vi "GPS显示界面.vi"() -> ()   [LabVIEW 2016, in "环境动力监测库.lvlib" / "NMEA.lvlib"]
uses:
  NMEA.lvlib
  NMEA_GPVTG-data.ctl
  NMEA_Mode.ctl
  NMEA_GPRMC-data.ctl
  NMEA_LatitudeDirection.ctl
  NMEA_LongitudeDirection.ctl
  NMEA_GPGGA-data.ctl
  NMEA_GPS-Quality.ctl
  <vilib>/Utility/miscctls.llb/LVPointTypeDef.ctl
  <vilib>/Utility/config.llb/NI_LVConfig.lvlib
panel:
  in  "解除告警":bool
  out "x+1":u32
  out "浮标定位点":cluster{"纬度":dbl, "经度":dbl} {"经度" format="%#.6g"; "纬度" format="%#.6g"}
  out "Port":string
  out "IP":string
  in  "手动设置定位":bool caption="定位自动获取OFF/手动设置ON"
  out "波特率":u32
  out "串口":string
  in  "移位报警设定值":dbl=1000.0
  out "GPS-Quality":T1
  out "定位状态":bool=TRUE
  in  "配置":bool
  out "Coordinates":picture
  in  "reset odometer":bool
  out "方位角 (deg)":dbl(knob) scale=0.0..360.0
  out "偏移量/米":dbl format="%#.2f"
  out "水平运动速度 (km/h)":dbl(knob) scale=0.0..180.0
  out "海拔":dbl format="%.2f"
  out "纬度":dbl format="%#.6g"
  out "经度":dbl format="%#.6g"
  out "时间":timestamp format="%<%H:%M:%S>T"
  out "日期":timestamp format="%<%Y/%m/%d>T"
  out "$GPGGA-message_OUT":T2={"TimeStamp"=timestamp(0 s since 1904-01-01), "Latitude"=0.0, "Latitude-Direction"=enum."", "Longitude"=1.0, "Longitude-Direction"=enum."", "GPS-Quality"=enum."GPS fix (SPS)", "Number of Satellites"=0, "Horizontal Dilution of Precision"=0.0, "Altitude above Mean-Sea-Level"=0.0, "Geoidal separation"=0.0, "Time since last DGPS update"=0.0, "DGPS reference station ID"=0} {"Time since last DGPS update" format="%.02f [s]"; "Geoidal separation" format="%.02f [m]"; "Altitude above Mean-Sea-Level" format="%.02f [m]"; "Horizontal Dilution of Precision" format="%.02f [HDOP]"; "Longitude" format="%0.4f [long]"; "Latitude" format="%.04f [lat]"; "TimeStamp" format="%<%.2X>T"}
  out "$GPRMC-message_OUT":T5={"TimeStamp"=timestamp(0 s since 1904-01-01), "Validity"=FALSE, "Latitude"=0.0, "Latitude-Direction"=enum."North", "Longitude"=0.0, "Longitude-Direction"=enum."East", "Speed in knots"=0.0, "True course"=0.0, "Date Stamp"=timestamp(0 s since 1904-01-01), "Magnetic Variation (East/West)"=0.0} {"Magnetic Variation (East/West)" format="%.02f [deg]"; "Date Stamp" format="%<%x>T"; "True course" format="%.02f [deg]"; "Speed in knots" format="%.02f [kts]"; "Longitude" format="%0.4f [long]"; "Latitude" format="%.04f [lat]"; "TimeStamp" format="%<%.2X>T"}
  out "$GPVTG-message_OUT":T6={"True Course over Ground"=0.0, "Magnetic Course over Ground"=0.0, "Speed over Ground in knots"=0.0, "Speed over Ground in km/h"=1.0, "Mode"=""} {"Speed over Ground in km/h" format="%.02f [km/h]"; "Speed over Ground in knots" format="%.02f [kts]"; "Magnetic Course over Ground" format="%.02f [deg]"; "True Course over Ground" format="%.02f [deg]"}
  out "Raw data GPS":string
  # "米"
  # "GPS监测"
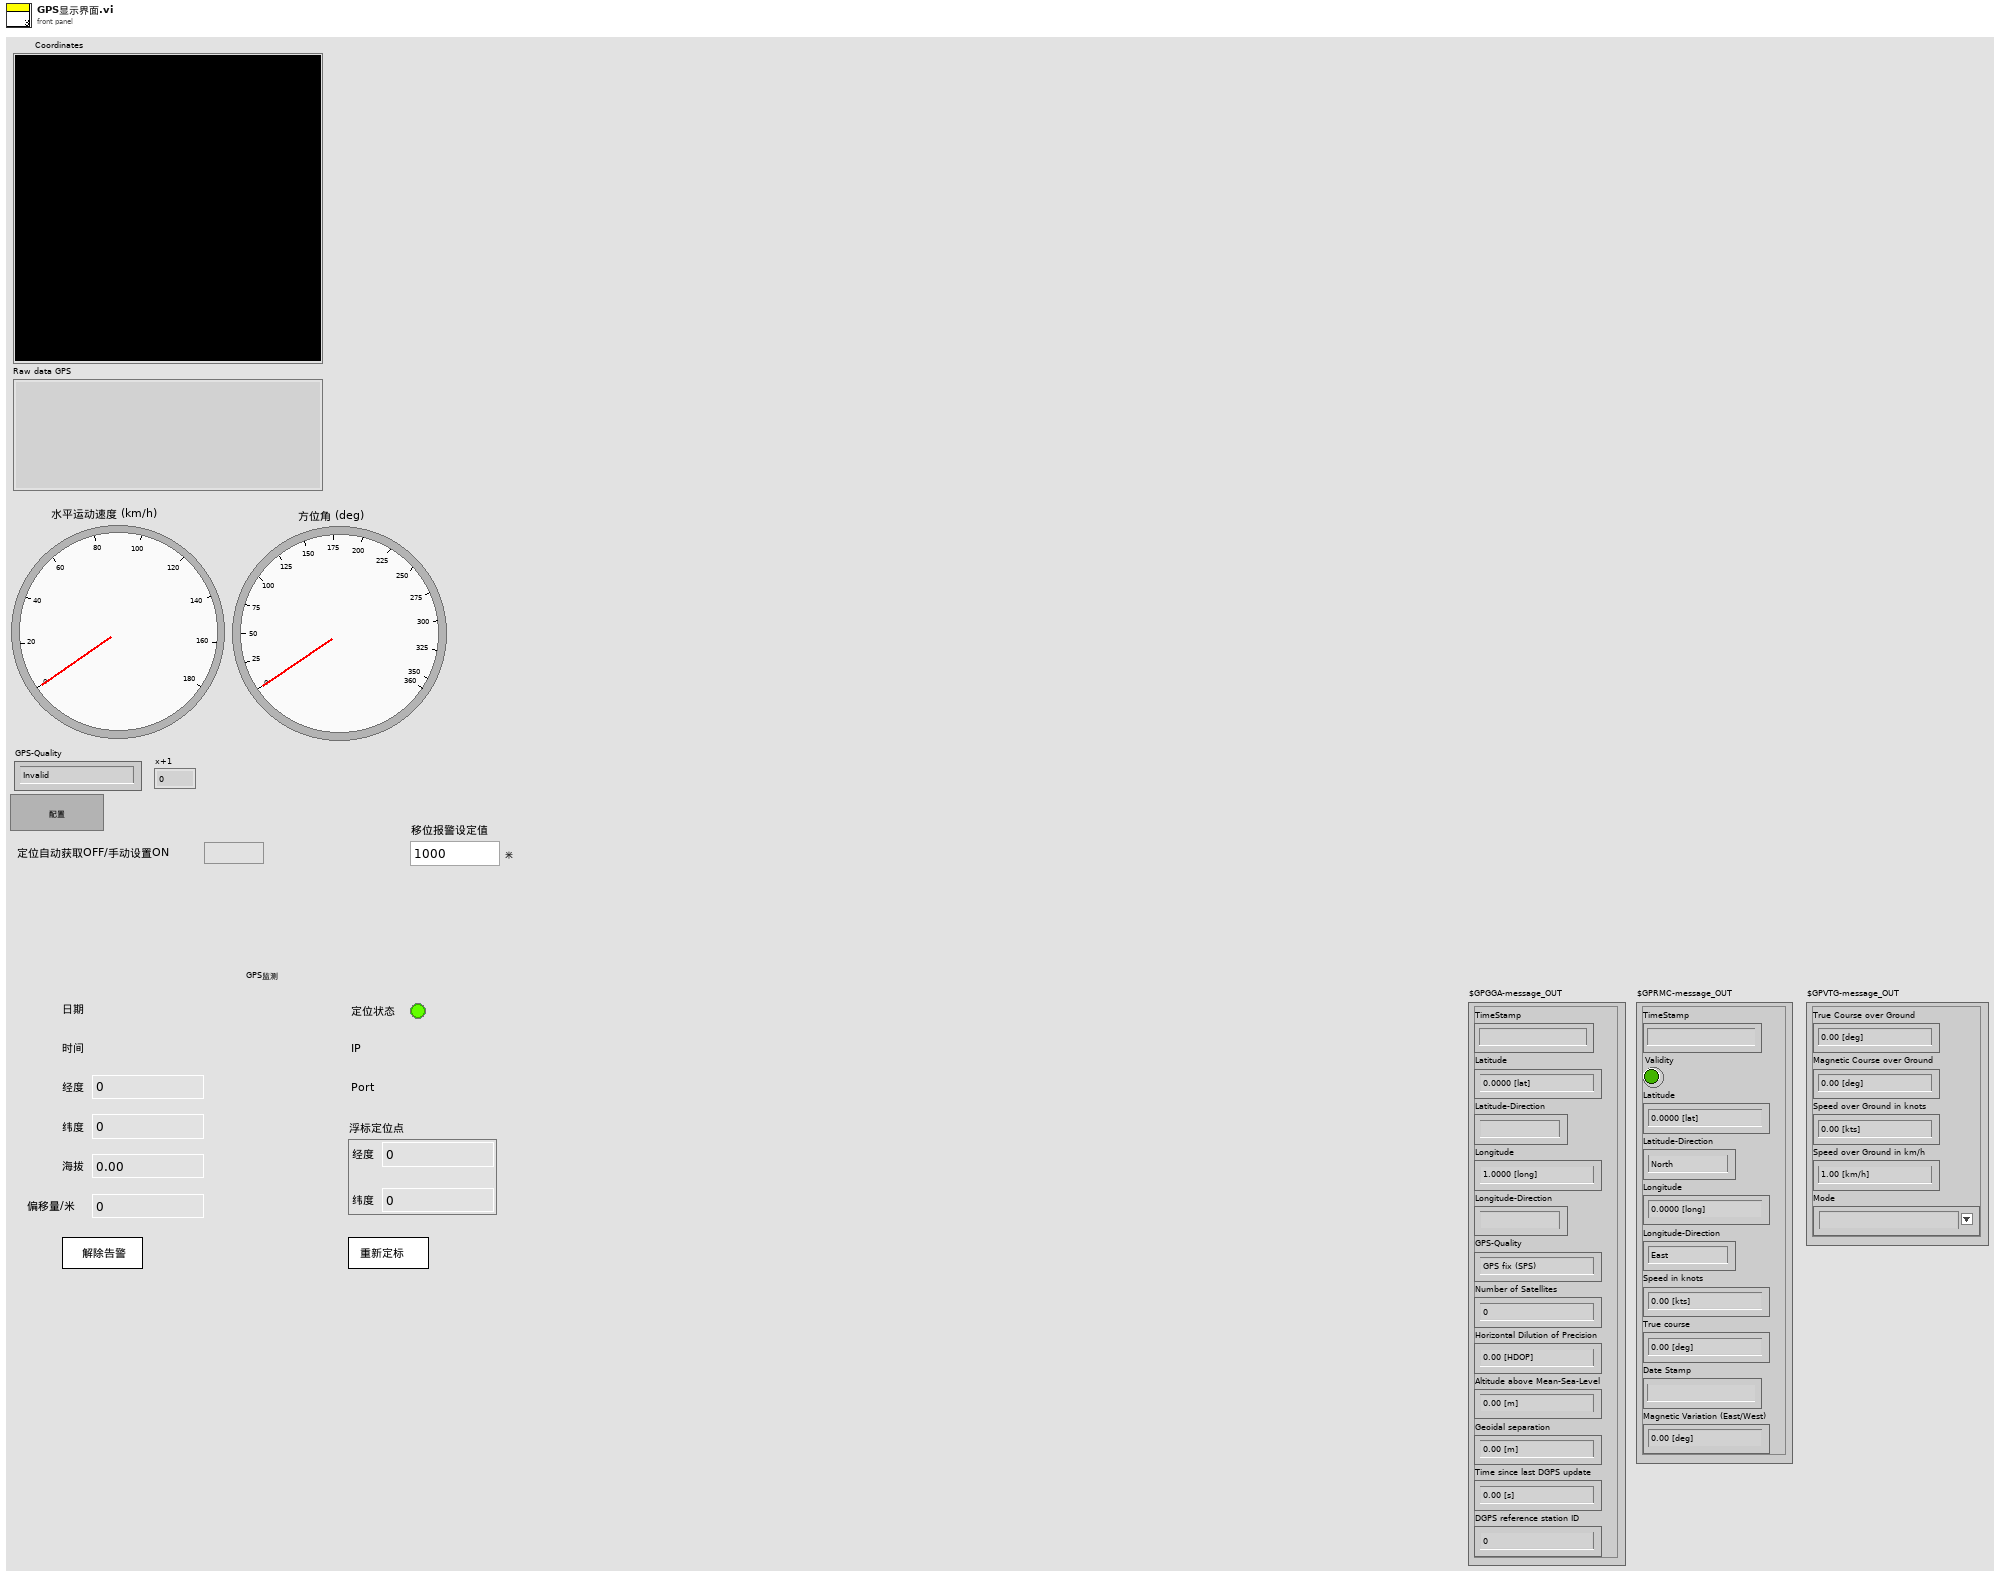
[diagram p1: front panel]
types:
  T1 = typedef "环境动力监测库.lvlib/NMEA.lvlib/NMEA_GPS-Quality.ctl" = enum16{"Invalid", "GPS fix (SPS)", "DGPS fix", "PPS fix", "Real Time Kinematic", "Float RTK", "estimated", "Manual input mode", "Simulation mode"}
  T2 = typedef "环境动力监测库.lvlib/NMEA.lvlib/NMEA_GPGGA-data.ctl" = cluster{"TimeStamp":timestamp, "Latitude":dbl, "Latitude-Direction":T3, "Longitude":dbl, "Longitude-Direction":T4, "GPS-Quality":T1, "Number of Satellites":i32, "Horizontal Dilution of Precision":dbl, "Altitude above Mean-Sea-Level":dbl, "Geoidal separation":dbl, "Time since last DGPS update":dbl, "DGPS reference station ID":i32}
  T3 = typedef "环境动力监测库.lvlib/NMEA.lvlib/NMEA_LatitudeDirection.ctl" = enum16{"", "North", "South"}
  T4 = typedef "环境动力监测库.lvlib/NMEA.lvlib/NMEA_LongitudeDirection.ctl" = enum16{"", "East", "West"}
  T5 = typedef "环境动力监测库.lvlib/NMEA.lvlib/NMEA_GPRMC-data.ctl" = cluster{"TimeStamp":timestamp, "Validity":bool, "Latitude":dbl, "Latitude-Direction":T3, "Longitude":dbl, "Longitude-Direction":T4, "Speed in knots":dbl, "True course":dbl, "Date Stamp":timestamp, "Magnetic Variation (East/West)":dbl}
  T6 = typedef "环境动力监测库.lvlib/NMEA.lvlib/NMEA_GPVTG-data.ctl" = cluster{"True Course over Ground":dbl, "Magnetic Course over Ground":dbl, "Speed over Ground in knots":dbl, "Speed over Ground in km/h":dbl, "Mode":T7}
  T7 = typedef "环境动力监测库.lvlib/NMEA.lvlib/NMEA_Mode.ctl" = string
  T8 = cluster{"监测项描述:输出":string, "连接方式":enum16{"串口", "TCP"}, "端口":string, "IP address:":string, "Port:":string, "站号":u64, "传感器型号":string, "波特率":u64, "data bits":u64, "停止位":u16, "奇偶校验":u16, "声光告警启用":bool}
  T9 = typedef "LVPointTypeDef.ctl" = cluster{"Horizontal":i16, "Vertical":i16}
  T10 = cluster{"定位状态":bool, "卫星数量":u16, "时间标识":timestamp, "纬度":dbl, "南北":string, "经度":dbl, "东西":string}
  T11 = cluster{"网络参数":cluster{"网络状态":bool, "本机IP":string[]}, "电源管理":cluster{"电源管理":bool, "氨氮电源":bool, "总磷电源":bool, "总氮电源":bool, "多参数电源":bool, "CODMn电源":bool, "CODCr电源":bool, "灯带电源":bool, "照明电源":bool}, "北斗-GPS":cluster{"GPS":cluster{"经度:":sgl, "纬度: ":sgl, "GPS监测":bool}, "北斗":cluster{"经度:":sgl, "纬度:":sgl, "北斗监测":bool}}}
  T12 = typedef "NI_LVConfig.lvlib/Config Data RefNum.ctl" = refnum<k1>
  T13 = cluster{"漏水监测输出":cluster{"漏水监测告警":bool, "告警内容":string}, "门禁监测输出":cluster{"门禁监测告警":bool, "告警内容":string}, "门禁监测输出2":cluster{"门禁监测告警":bool, "告警内容":string}, "温湿度监测输出":cluster{"温湿度监测告警":bool, "告警内容":string}, "烟雾监测输出":cluster{"烟雾监测告警":bool, "告警内容":string}, "空调监测输出":cluster{"空调监测告警":bool, "告警内容":string}, "自动重合闸输出":cluster{"自动重合闸告警":bool, "告警内容":string}, "红外入侵输出":cluster{"红外入侵告警":bool, "告警内容":string}, "振动输出":cluster{"振动告警":bool, "告警内容":string}, "UPS输出":cluster{"UPS告警":bool, "告警内容":string}, "蓄电池输出":cluster{"蓄电池告警":bool, "告警内容":string}, "蓄电池输出2":cluster{"蓄电池告警":bool, "告警内容":string}, "GPS输出":cluster{"定位告警":bool, "告警内容":string}, "北斗输出":cluster{"定位告警":bool, "告警内容":string}, "气象输出":cluster{"气象告警":bool, "告警内容":string}}
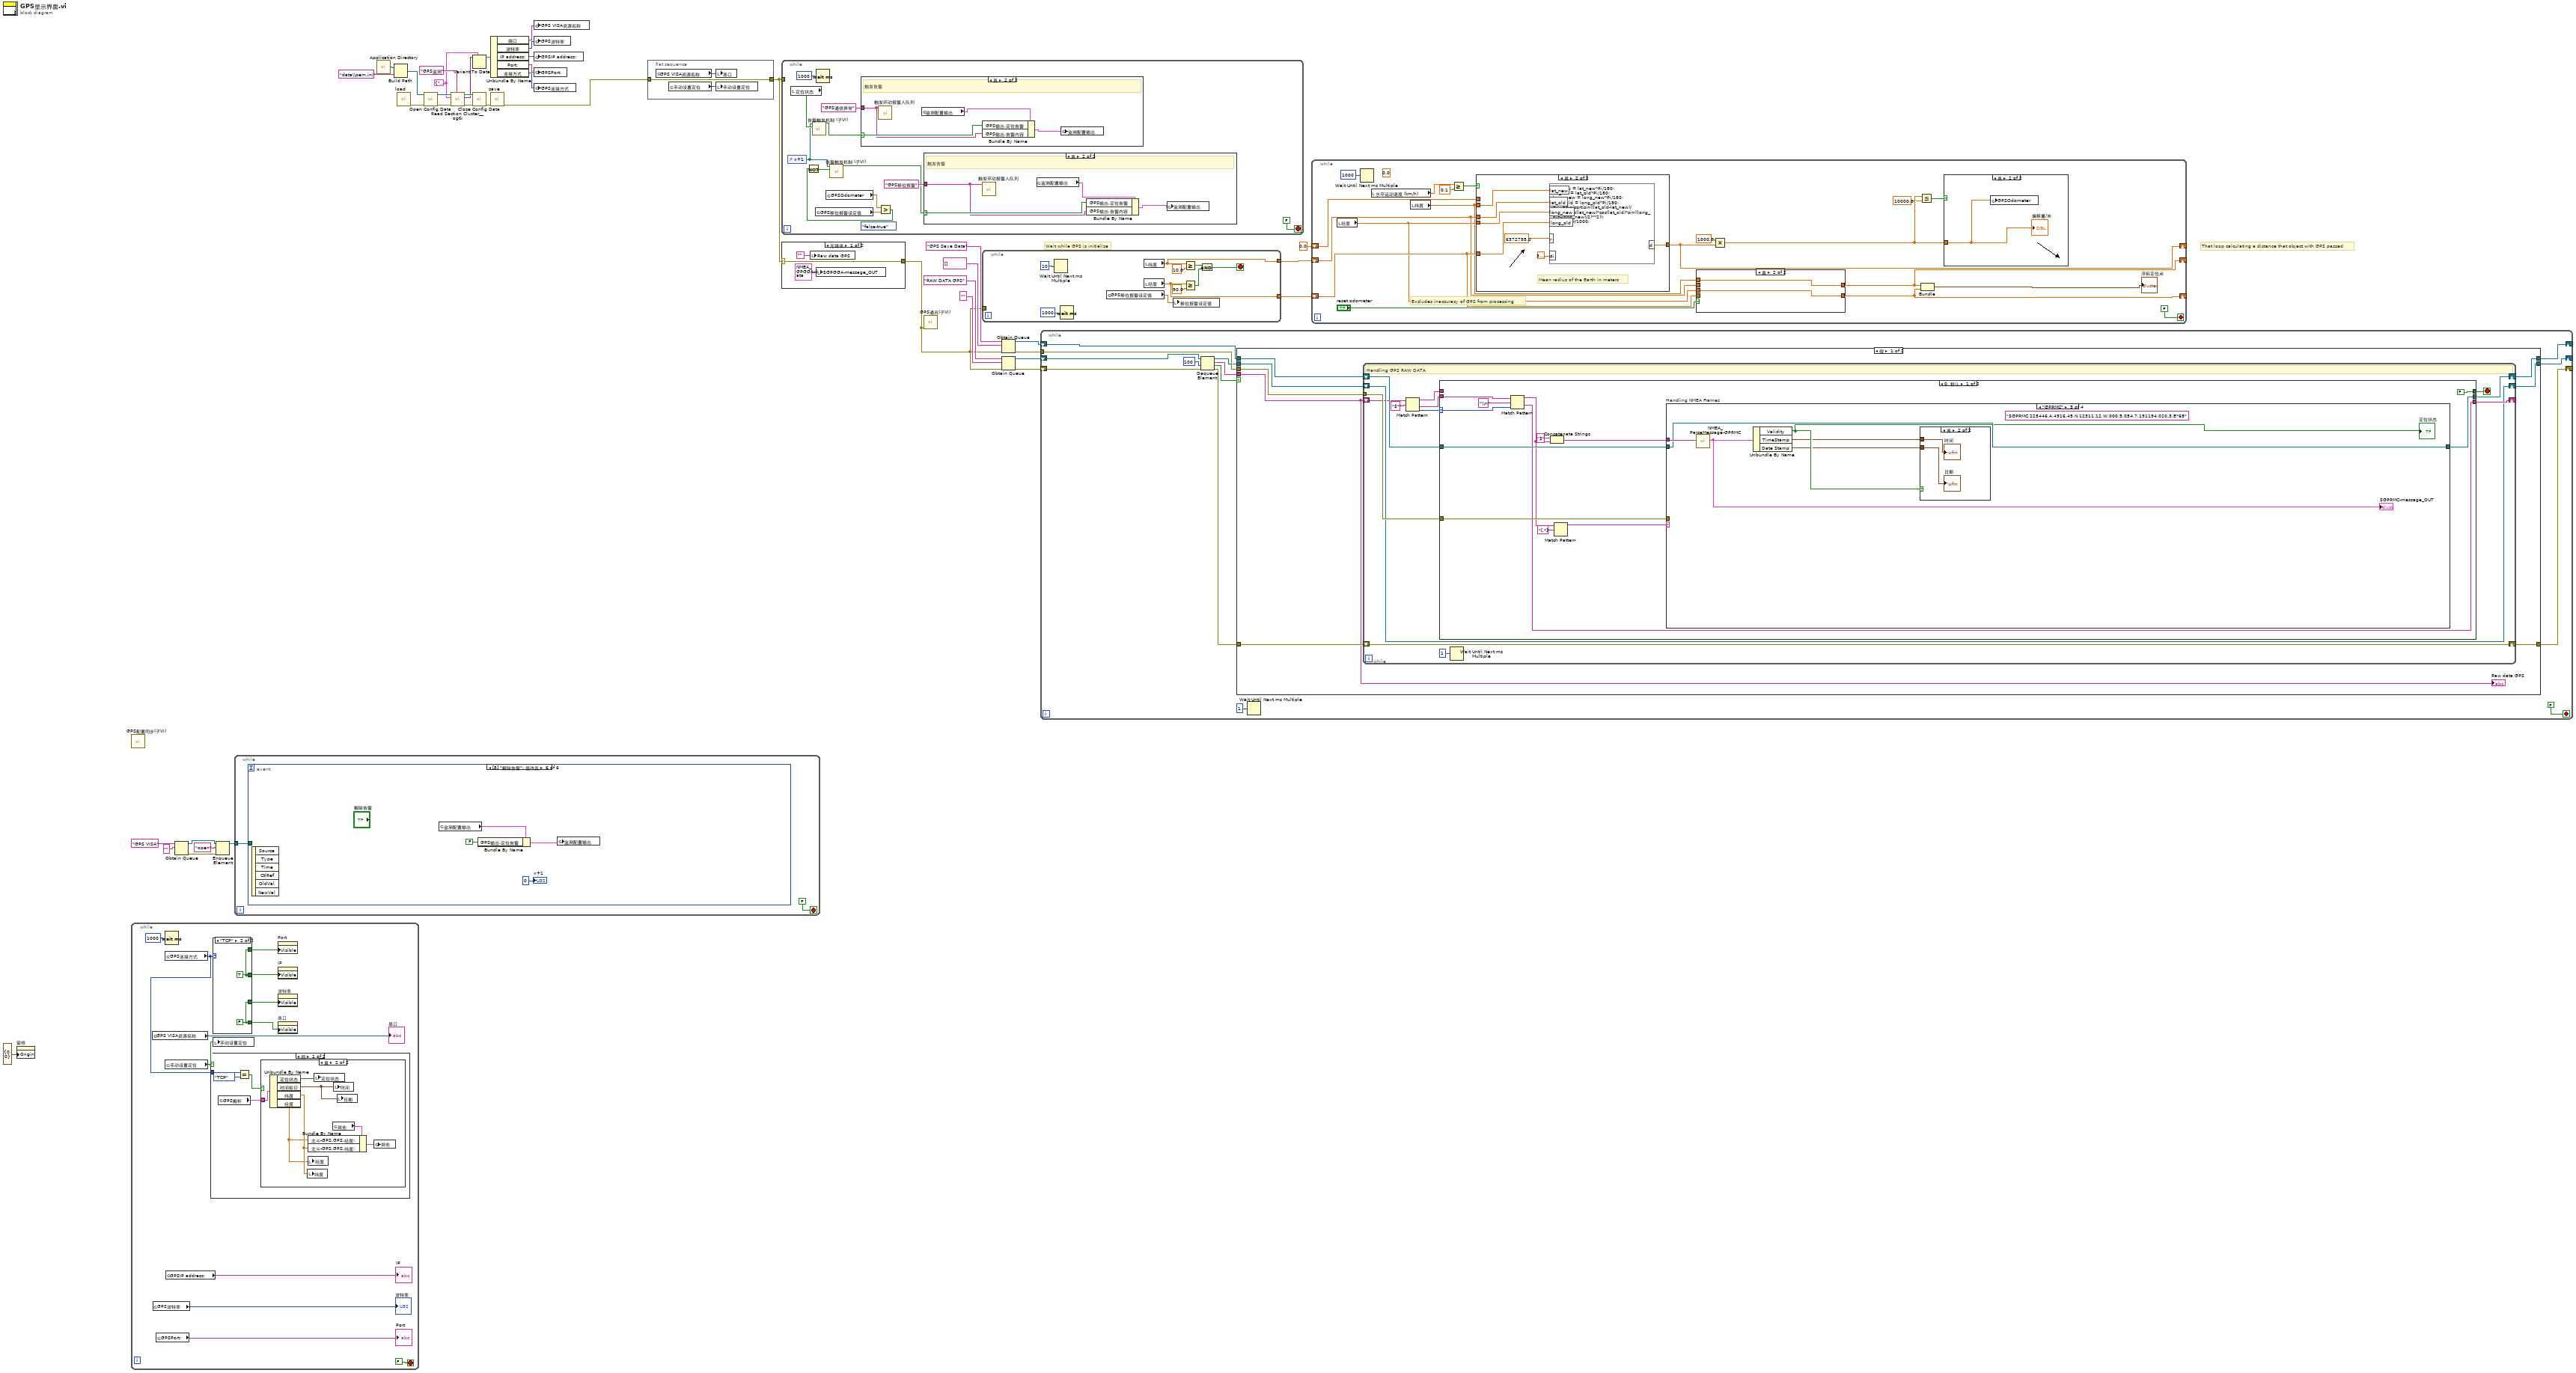
[diagram p0: block diagram]
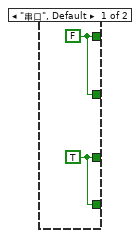
[diagram p4: hidden frame]
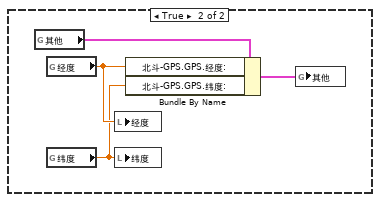
[diagram p6: hidden frame]
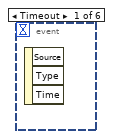
[diagram p7: hidden frame]
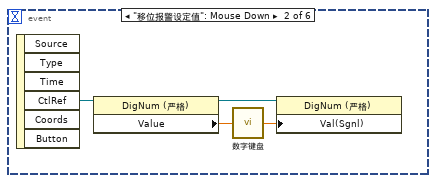
[diagram p8: hidden frame]
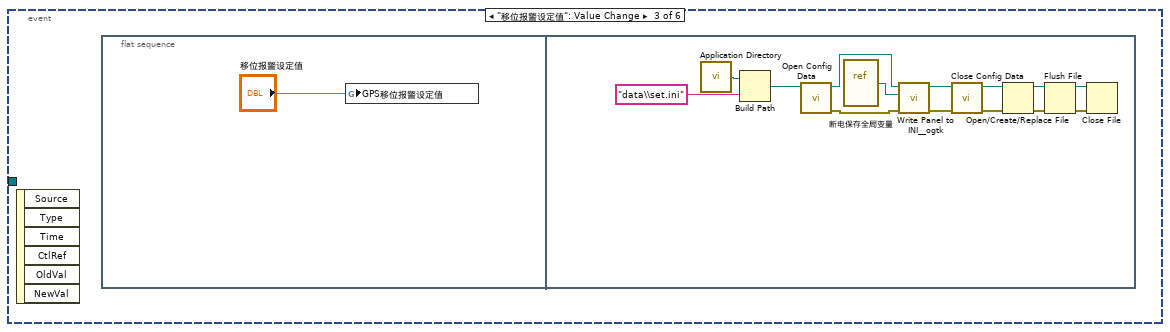
[diagram p9: hidden frame]
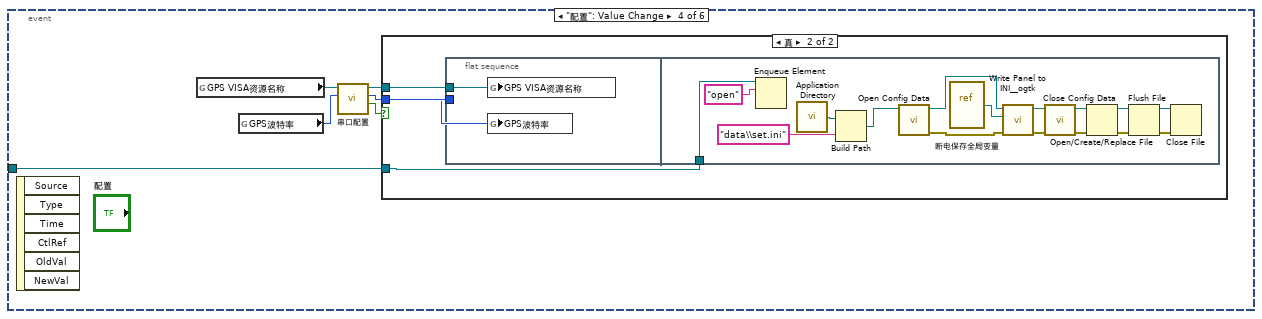
[diagram p10: hidden frame]
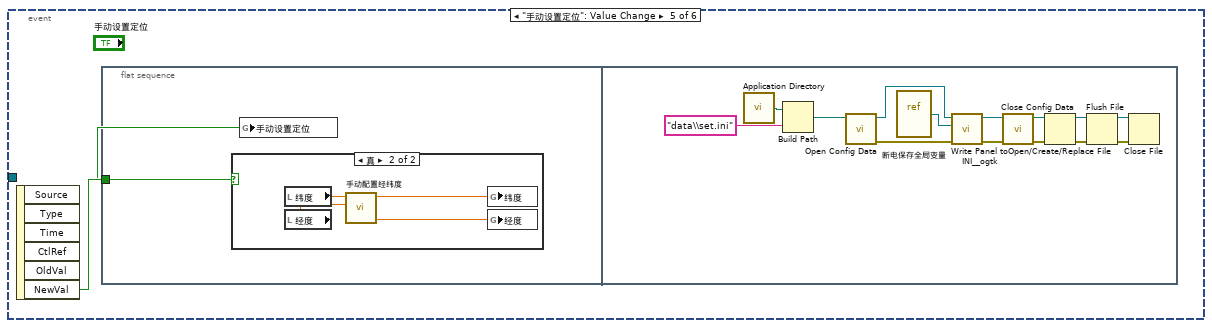
[diagram p12: hidden frame]
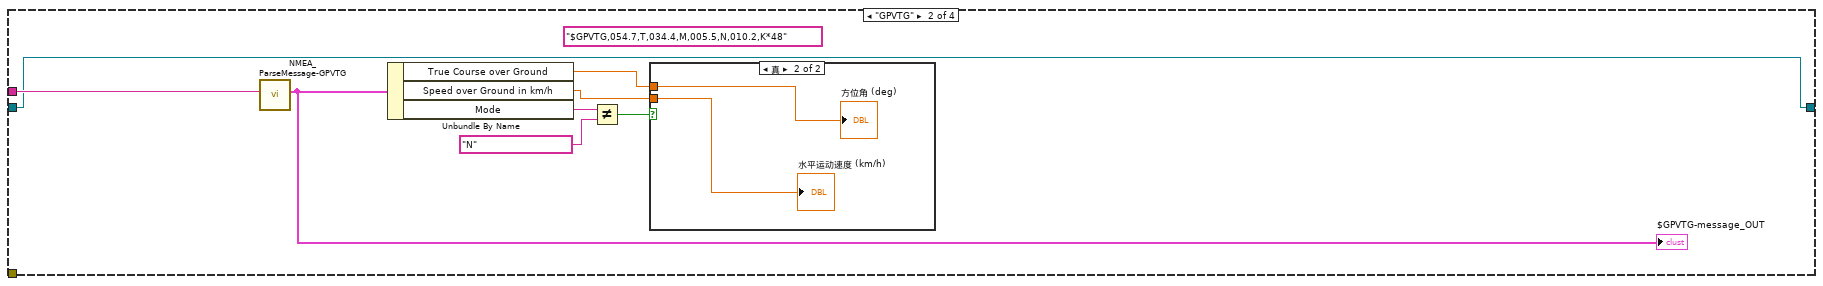
[diagram p19: hidden frame]
diagram:
  w9 = T8 {"监测项描述:输出"="", "连接方式"=enum."串口", "端口"="", "IP address:"="", "Port:"="", "站号"=19200, "传感器型号"="", "波特率"=19200, "data bits"=8, "停止位"=10, "奇偶校验"=0, "声光告警启用"=FALSE} ("输入簇")
  (unwired) 0.0 ("方位角 (deg)")
  # "That loop calculating a distance that object with GPS passed"
  # "Wait while GPS is initialize"
  n1 = property on="窗格" class="Pane"("Origin"=T9 {"Horizontal"=0, "Vertical"=0} ("原点")) -> ()  [unwired: 2 in, 2 out]
  n2 = call "GPS配置同步(子VI).vi"() -> ()  [unwired: 12 in]
  n3 = while {
    stop <- FALSE stop-if-true
    n4 = global read "断电保存全局变量.vi" "GPS VISA资源名称"() -> (→"串口":refnum<visa-resource-name>)
    n5 = global read "断电保存全局变量.vi" "GPS波特率"() -> (→"波特率":u32)
    n6 = global read "断电保存全局变量.vi" "GPSPort:"() -> (→"Port":string)
    n7 = Wait (ms)(milliseconds to wait=u32 1000 ("等待时间（毫秒）")) -> ()  [unwired: 1 out]
    n8 = global read "断电保存全局变量.vi" "GPS连接方式"() -> (w40:enum16{"串口", "TCP"})
    n9 = global read "断电保存全局变量.vi" "手动设置定位"() -> (w47:bool)
    n10 = global read "断电保存全局变量.vi" "GPSIP address:"() -> (→"IP":string)
    n11 = case shown="假" w47 {
      tunnel: w40 -> [w59 _]
      frame False {
        n12 = global read "NMEA过程全局变量.vi" "GPS解析"() -> (w56:T10)
        n13 = Equal?(x=w59, y=enum16{"串口", "TCP"}."TCP") -> (x = y?=w57:bool)
        n14 = case shown="真" w57 {
          tunnel: w56 -> [_ w66]
          frame False {
          }
          frame True {
            n15 = Unbundle By Name(w66) -> ("定位状态"=w65:bool, "时间标识"=w64:timestamp, "纬度"=w61:dbl, "经度"=w60:dbl)
            n16 = local write "纬度"(w61) -> ()
            n17 = local write "经度"(w60) -> ()
            n18 = local write "定位状态"(w65) -> ()
            n19 = global read "内部交互全局变量.vi" "其他"() -> (w63:T11)
            n20 = Bundle By Name(cluster=w63, "北斗-GPS.GPS.经度:"=w60, "北斗-GPS.GPS.纬度:"=w61) -> (w62:T11)
            n21 = local write "时间"(w64) -> ()
            n22 = local write "日期"(w64) -> ()
            n23 = global write "内部交互全局变量.vi" "其他"(w62) -> ()
          }
        }
      }
      frame True {
        n24 = global read "内部交互全局变量.vi" "其他"() -> (w70:T11)
        n25 = global read "断电保存全局变量.vi" "经度"() -> (w68:dbl)
        n26 = global read "断电保存全局变量.vi" "纬度"() -> (w67:dbl)
        n27 = local write "经度"(w68) -> ()
        n28 = local write "纬度"(w67) -> ()
        n29 = Bundle By Name(cluster=w70, "北斗-GPS.GPS.经度:"=w68, "北斗-GPS.GPS.纬度:"=w67) -> (w69:T11)
        n30 = global write "内部交互全局变量.vi" "其他"(w69) -> ()
      }
    }
    n31 = case shown="\"TCP\"" w40 {
      tunnel: [w53 w55] -> w44
      tunnel: [w53 w55] -> w43
      tunnel: [w52 w54] -> w42
      tunnel: [w52 w54] -> w41
      frame "串口", Default {
        w52 = FALSE
        w53 = TRUE
      }
      frame "TCP" {
        w54 = TRUE
        w55 = FALSE
      }
    }
    n32 = local write "手动设置定位"(w47) -> ()
    n33 = property on="Port" class="Str"("Visible"=w41) -> ()  [unwired: 2 in, 2 out]
    n34 = property on="IP" class="Str"("Visible"=w42) -> ()  [unwired: 2 in, 2 out]
    n35 = property on="波特率" class="DigNum (严格)"("Visible"=w43) -> ()  [unwired: 2 in, 2 out]
    n36 = property on="串口" class="Str"("Visible"=w44) -> ()  [unwired: 2 in, 2 out]
  }
  n37 = Obtain Queue(name (unnamed)="GPS VISA" ("名称（未命名）"), element data type="" ("名称（未命名）")) -> (queue out=w24:refnum<queue>, error out=w23:errorcluster)  [unwired: 3 in, 1 out]
  n38 = Enqueue Element(queue=w24, element="open" ("元素"), error in (no error)=w23) -> (queue out=w21:refnum<queue>)  [unwired: 1 in, 2 out]
  n39 = while {
    tunnel: w21 -> [w72]
    stop <- FALSE stop-if-true
    n40 = event shown="[5] \"解除告警\": 值改变" {
      selector: _ -> [_ _ _ _ _ _]
      dyn-events: _ -> [_ _ _ _ _ _]
      timeout: _ -> [_ _ _ _ _ _]
      tunnel: w72 -> [_ _ _ w92 _ _]
      event Timeout {
        n41 = event-data() -> ()  [unwired: 1 in, 3 out]
      }
      event "移位报警设定值": Mouse Down {
        n42 = event-data() -> ("CtlRef"=w73:refnum<vi>)  [unwired: 1 in, 5 out]
        n43 = property class="DigNum (严格)"(reference=w73) -> (reference out=w74:refnum<vi>, "Value"=w76:dbl)  [unwired: 1 in, 1 out]
        n44 = call "数字键盘.vi"("OldNumber"=w76) -> ("NewNumber"=w75:dbl)
        n45 = property class="DigNum (严格)"(reference=w74, "Val(Sgnl)"=w75) -> ()  [unwired: 1 in, 2 out]
      }
      event "移位报警设定值": Value Change {
        n46 = event-data() -> ()  [unwired: 1 in, 6 out]
        n47 = flat-sequence {
          frame #0 {
            n48 = global write "断电保存全局变量.vi" "GPS移位报警设定值"("移位报警设定值") -> ()
          }
          frame #1 {
            n49 = call <vilib>:"Application Directory.vi"() -> ("Application Directory"=w90:path)
            n50 = Build Path(base path=w90, name or relative path="data\\set.ini" ("名称或相对路径")) -> (appended path=w91:path)
            n51 = call <vilib>:"Open Config Data.vi"("configuration file path"=w91) -> ("error out"=w87:errorcluster, "refnum"=w88:T12)  [unwired: 8 in, 1 out]
            n52 = vi-ref "断电保存全局变量.vi"() -> (w84:refnum<vi>)
            n53 = call <userlib>:"Write Panel to INI__ogtk.vi"("error in (no error)"=w87, "VI ref"=w84, "refnum"=w88) -> ("error out"=w85:errorcluster, "refnum out"=w86:T12)  [unwired: 7 in]
            n54 = call <vilib>:"Close Config Data.vi"("error in (no error)"=w85, "refnum"=w86) -> ("error out"=w83:errorcluster, "file path"=w82:path)  [unwired: 8 in]
            n55 = Open/Create/Replace File(file path (use dialog)=w82, error in=w83) -> (refnum out=w80:refnum<file>, error out=w81:errorcluster)  [unwired: 4 in, 1 out]
            n56 = Flush File(refnum=w80, error in=w81) -> (refnum out=w78:refnum<file>, error out=w79:errorcluster)
            n57 = Close File(refnum=w78, error in=w79) -> ()  [unwired: 2 out]
          }
        }
      }
      event "配置": Value Change {
        n58 = event-data() -> ()  [unwired: 1 in, 6 out]
        n59 = global read "断电保存全局变量.vi" "GPS VISA资源名称"() -> (w95:refnum<visa-resource-name>)
        n60 = global read "断电保存全局变量.vi" "GPS波特率"() -> (w93:u32)
        n61 = call "串口配置.vi"("波特率"=w93, "VISA资源名称"=w95) -> ("确认 2"=w97:bool, "波特率输出"=w94:u32, "VISA资源名称 2"=w96:refnum<visa-resource-name>)  [unwired: 7 in]
        n62 = case shown="真" w97 {
          tunnel: w96 -> [_ w100]
          tunnel: w94 -> [_ w99]
          tunnel: w92 -> [_ w98]
          frame False {
          }
          frame True {
            n63 = flat-sequence {
              tunnel: w100 -> [w102]
              tunnel: w99 -> [w101]
              tunnel: w98 -> [w104]
              frame #0 {
                n64 = global write "断电保存全局变量.vi" "GPS VISA资源名称"(w102) -> ()
                n65 = global write "断电保存全局变量.vi" "GPS波特率"(w101) -> ()
              }
              frame #1 {
                n66 = Enqueue Element(queue=w104, element="open" ("元素")) -> ()  [unwired: 2 in, 3 out]
                n67 = call <vilib>:"Application Directory.vi"() -> ("Application Directory"=w117:path)
                n68 = Build Path(base path=w117, name or relative path="data\\set.ini" ("名称或相对路径")) -> (appended path=w118:path)
                n69 = call <vilib>:"Open Config Data.vi"("configuration file path"=w118) -> ("error out"=w114:errorcluster, "refnum"=w115:T12)  [unwired: 8 in, 1 out]
                n70 = vi-ref "断电保存全局变量.vi"() -> (w111:refnum<vi>)
                n71 = call <userlib>:"Write Panel to INI__ogtk.vi"("error in (no error)"=w114, "VI ref"=w111, "refnum"=w115) -> ("error out"=w112:errorcluster, "refnum out"=w113:T12)  [unwired: 7 in]
                n72 = call <vilib>:"Close Config Data.vi"("error in (no error)"=w112, "refnum"=w113) -> ("error out"=w110:errorcluster, "file path"=w109:path)  [unwired: 8 in]
                n73 = Open/Create/Replace File(file path (use dialog)=w109, error in=w110) -> (refnum out=w107:refnum<file>, error out=w108:errorcluster)  [unwired: 4 in, 1 out]
                n74 = Flush File(refnum=w107, error in=w108) -> (refnum out=w105:refnum<file>, error out=w106:errorcluster)
                n75 = Close File(refnum=w105, error in=w106) -> ()  [unwired: 2 out]
              }
            }
          }
        }
      }
      event "手动设置定位": Value Change {
        n76 = event-data() -> ("NewVal"=w119:bool)  [unwired: 1 in, 5 out]
        n77 = flat-sequence {
          tunnel: w119 -> [w120]
          frame #0 {
            n78 = case shown="真" w120 {
              frame False {
              }
              frame True {
                n79 = local read "纬度"() -> (w124:dbl)
                n80 = local read "经度"() -> (w123:dbl)
                n81 = call "手动配置经纬度.vi"("经度输入"=w123, "纬度输入"=w124) -> ("经度"=w121:dbl, "纬度"=w122:dbl)  [unwired: 8 in]
                n82 = global write "断电保存全局变量.vi" "纬度"(w122) -> ()
                n83 = global write "断电保存全局变量.vi" "经度"(w121) -> ()
              }
            }
            n84 = global write "断电保存全局变量.vi" "手动设置定位"(w120) -> ()
          }
          frame #1 {
            n85 = call <vilib>:"Application Directory.vi"() -> ("Application Directory"=w137:path)
            n86 = Build Path(base path=w137, name or relative path="data\\set.ini" ("名称或相对路径")) -> (appended path=w138:path)
            n87 = call <vilib>:"Open Config Data.vi"("configuration file path"=w138) -> ("error out"=w134:errorcluster, "refnum"=w135:T12)  [unwired: 8 in, 1 out]
            n88 = vi-ref "断电保存全局变量.vi"() -> (w131:refnum<vi>)
            n89 = call <userlib>:"Write Panel to INI__ogtk.vi"("error in (no error)"=w134, "VI ref"=w131, "refnum"=w135) -> ("error out"=w132:errorcluster, "refnum out"=w133:T12)  [unwired: 7 in]
            n90 = call <vilib>:"Close Config Data.vi"("error in (no error)"=w132, "refnum"=w133) -> ("error out"=w130:errorcluster, "file path"=w129:path)  [unwired: 8 in]
            n91 = Open/Create/Replace File(file path (use dialog)=w129, error in=w130) -> (refnum out=w127:refnum<file>, error out=w128:errorcluster)  [unwired: 4 in, 1 out]
            n92 = Flush File(refnum=w127, error in=w128) -> (refnum out=w125:refnum<file>, error out=w126:errorcluster)
            n93 = Close File(refnum=w125, error in=w126) -> ()  [unwired: 2 out]
          }
        }
      }
      event "解除告警": Value Change {
        n94 = event-data() -> ()  [unwired: 1 in, 6 out]
        n95 = global read "内部交互全局变量.vi" "监测配置输出"() -> (w140:T13)
        n96 = Bundle By Name(cluster=w140, "GPS输出.定位告警"=FALSE) -> (w139:T13)
        n97 = global write "内部交互全局变量.vi" "监测配置输出"(w139) -> ()
        "x+1" <- u32 0 ("x+1")
      }
    }
  }
  n98 = call <vilib>:"Application Directory.vi"() -> ("Application Directory"=w16:path)
  n99 = Build Path(base path=w16, name or relative path="data\\pem.ini" ("名称或相对路径")) -> (appended path=w17:path)
  n100 = call "load.vi"() -> ("error out"=w3:errorcluster)  [unwired: 11 in]
  n101 = call <vilib>:"Open Config Data.vi"("error in (no error)"=w3, "configuration file path"=w17) -> ("error out"=w18:errorcluster, "refnum"=w19:T12)  [unwired: 7 in, 1 out]
  n102 = call <userlib>:"Read Section Cluster__ogtk.vi"("section (optional)"="GPS监测", "error in (no error)"=w18, "Section Formatted Cluster Type"=w9, "refnum"=w19) -> ("error out"=w12:errorcluster, "Section Formatted Cluster"=w11:variant, "dup refnum"=w13:T12)  [unwired: 3 in, 2 out]
  n103 = Variant To Data(type=w9, Variant=w11) -> (data=w10:T8)  [unwired: 1 in, 1 out]
  n104 = call <vilib>:"Close Config Data.vi"("error in (no error)"=w12, "refnum"=w13) -> ("error out"=w2:errorcluster)  [unwired: 8 in, 1 out]
  n105 = Unbundle By Name(w10) -> ("端口"=w8:string, "波特率"=w7:u64, "IP address:"=w6:string, "Port:"=w5:string, "连接方式"=w4:enum16{"串口", "TCP"})
  n106 = call "save.vi"("error in (no error)"=w2) -> ("error out"=w1:errorcluster)  [unwired: 10 in]
  n107 = global write "断电保存全局变量.vi" "GPS VISA资源名称"(w8) -> ()
  n108 = global write "断电保存全局变量.vi" "GPS波特率"(w7) -> ()
  n109 = global write "断电保存全局变量.vi" "GPSIP address:"(w6) -> ()
  n110 = global write "断电保存全局变量.vi" "GPSPort:"(w5) -> ()
  n111 = global write "断电保存全局变量.vi" "GPS连接方式"(w4) -> ()
  n112 = flat-sequence {
    tunnel: w1 -> [w144]
    tunnel: [w144] -> w27
    frame #0 {
      n113 = global read "断电保存全局变量.vi" "GPS VISA资源名称"() -> (w145:refnum<visa-resource-name>)
      n114 = global read "断电保存全局变量.vi" "手动设置定位"() -> (w143:bool)
      n115 = local write "串口"(w145) -> ()
      n116 = local write "手动设置定位"(w143) -> ()
    }
  }
  n117 = while {
    tunnel: w27 -> [_]
    stop <- FALSE stop-if-true
    (unwired) enum16{"either", "false-true", "true-false"}."false-true" ("direction")
    n118 = control-ref of="x+1"() -> (w147:refnum<vi>)
    n119 = local read "定位状态"() -> (w148:bool)
    n120 = call "告警触发机制 (子VI).vi"("状态输出"=w148, "Digital输入"=w147) -> ("触发告警"=w146:bool)  [unwired: 8 in, 1 out]
    n121 = global read "断电保存全局变量.vi" "GPS移位报警设定值"() -> (w155:dbl)
    n122 = Wait (ms)(milliseconds to wait=u32 1000 ("等待时间（毫秒）")) -> ()  [unwired: 1 out]
    n123 = global read "NMEA过程全局变量.vi" "GPSOdometer"() -> (w156:dbl)
    n124 = case shown="真" w146 {
      selector: w146 -> [_ w161]
      tunnel: "GPS通信异常" ("设备") -> [_ w160]
      frame False {
      }
      frame True {
        # "触发告警"
        n125 = call "触发环动报警入队列.vi"("报警内容"=w160) -> ()  [unwired: 11 in]
        n126 = global read "内部交互全局变量.vi" "监测配置输出"() -> (w159:T13)
        n127 = Bundle By Name(cluster=w159, "GPS输出.定位告警"=w161, "GPS输出.告警内容"=w160) -> (w158:T13)
        n128 = global write "内部交互全局变量.vi" "监测配置输出"(w158) -> ()
      }
    }
    n129 = Greater?(x=w156, y=w155) -> (0:w150:bool)
    n130 = Not(x=w150) -> (.not. x?=w151:bool)
    n131 = call "告警触发机制 (子VI).vi"("状态输出"=w151, "Digital输入"=w147) -> ("触发告警"=w149:bool)  [unwired: 8 in, 1 out]
    n132 = case shown="真" w149 {
      selector: w149 -> [_ w165]
      tunnel: "GPS移位报警" ("设备") -> [_ w164]
      frame False {
      }
      frame True {
        # "触发告警"
        n133 = call "触发环动报警入队列.vi"("报警内容"=w164) -> ()  [unwired: 11 in]
        n134 = global read "内部交互全局变量.vi" "监测配置输出"() -> (w163:T13)
        n135 = Bundle By Name(cluster=w163, "GPS输出.定位告警"=w165, "GPS输出.告警内容"=w164) -> (w162:T13)
        n136 = global write "内部交互全局变量.vi" "监测配置输出"(w162) -> ()
      }
    }
  }
  n137 = case shown="无错误" w27 {
    selector: w27 -> [w167 w169]
    tunnel: [w167 w169] -> w20
    frame No Error {
      n138 = local write "Raw data GPS"("") -> ()
      n139 = local write "$GPGGA-message_OUT"(T2 {"TimeStamp"=timestamp(0 s since 1904-01-01), "Latitude"=0.0, "Latitude-Direction"=enum."North", "Longitude"=0.0, "Longitude-Direction"=enum."East", "GPS-Quality"=enum."Invalid", "Number of Satellites"=0, "Horizontal Dilution of Precision"=0.0, "Altitude above Mean-Sea-Level"=0.0, "Geoidal separation"=0.0, "Time since last DGPS update"=0.0, "DGPS reference station ID"=0} ("GPGGA-data")) -> ()
    }
    frame Error {
    }
  }
  n140 = call "GPS通讯(子VI).vi"("error in (no error)"=w20) -> ()  [unwired: 11 in]
  n141 = while {
    tunnel: [w174] -> w29
    tunnel: [w176] -> w30
    tunnel: w20 -> [_]
    stop <- w170 stop-if-true
    n142 = Wait Until Next ms Multiple(millisecond multiple=u32 10) -> ()  [unwired: 1 out]
    n143 = Wait (ms)(milliseconds to wait=u32 1000 ("等待时间（毫秒）")) -> ()  [unwired: 1 out]
    n144 = global read "断电保存全局变量.vi" "GPS移位报警设定值"() -> (w178:dbl)
    n145 = local read "纬度"() -> (w176:dbl)
    n146 = local read "经度"() -> (w174:dbl)
    n147 = local write "移位报警设定值"(w178) -> ()
    n148 = Greater Or Equal?(x=w176, y=10.0) -> (x >= y?=w171:bool)
    n149 = Greater Or Equal?(x=w174, y=90.0) -> (x >= y?=w172:bool)
    n150 = And(x=w171, y=w172) -> (x .and. y?=w170:bool)
  }
  n151 = Obtain Queue(name (unnamed)="GPS Save Data" ("名称（未命名）"), element data type=string[] [], error in (no error)=w20) -> (queue out=w38:refnum<queue>, error out=w37:errorcluster)  [unwired: 2 in, 1 out]
  n152 = Obtain Queue(name (unnamed)="RAW DATA GPS" ("nom (aucun)"), element data type="" ("expression régulière"), error in (no error)=w20) -> (queue out=w35:refnum<queue>, error out=w39:errorcluster)  [unwired: 2 in, 1 out]
  n153 = while {
    tunnel: w37 -> [w189]
    shift-right: [w187] -> _
    shift-left: w35 -> [w188]
    shift-right: [w183] -> _
    shift-left: w38 -> [w190]
    shift-right: [w182] -> _
    shift-left: w39 -> [w193]
    stop <- FALSE stop-if-true
    n154 = Dequeue Element(queue=w188, timeout in ms (-1)=100 ("timeout en ms (-1)"), error in (no error)=w193) -> (queue out=w186:refnum<queue>, element=w192:string, timed out?=w184:bool, error out=w181:errorcluster)
    n155 = case shown="假" w184 {
      tunnel: w192 -> [w194 _]
      tunnel: w190 -> [w201 w296]
      tunnel: w189 -> [w200 _]
      tunnel: [w199 w297] -> w187
      tunnel: w186 -> [w198 w297]
      tunnel: [w197 w296] -> w183
      tunnel: [w196 w295] -> w182
      tunnel: w181 -> [w195 w295]
      frame False {
        n156 = while {
          shift-right: [w212] -> _
          shift-left: w194 -> [w203]
          tunnel: w200 -> [w208]
          shift-right: [w207] -> w199
          shift-left: w198 -> [w207]
          shift-right: [w205] -> w197
          shift-left: w201 -> [w209]
          shift-right: [w204] -> w196
          shift-left: w195 -> [w204]
          stop <- w206 stop-if-true
          # "Handling GPS RAW DATA"
          n157 = Match Pattern(string=w203, regular expression="$*" ("expression régulière")) -> (before substring=w202:string, after substring=w211:string, offset past match=w213:i32)  [unwired: 1 in, 1 out]
          n158 = case shown="0, 默认" w213 {
            selector: w213 -> [w226 _]
            tunnel: [w225 w292] -> w212
            tunnel: w211 -> [w227 _]
            tunnel: [FALSE TRUE] -> w206
            tunnel: w209 -> [w221 w293]
            tunnel: w208 -> [w220 _]
            tunnel: [w218 w293] -> w205
            tunnel: w202 -> [_ w292]
            frame 0, Default {
              n159 = Match Pattern(string=w227, regular expression="\\n" ("expression régulière"), offset (0)=w226) -> (before substring=w217:string, after substring=w225:string)  [unwired: 2 out]
              n160 = Concatenate Strings("$" ("expression régulière"), w217) -> (w223:string)
              n161 = Match Pattern(string=w217, regular expression="[,*]" ("正则表达式")) -> (before substring=w215:string)  [unwired: 1 in, 3 out]
              n162 = case "Handling NMEA Frames" shown="\"GPRMC\"" w215 {
                tunnel: w223 -> [_ w236 w244 w265]
                tunnel: w221 -> [w228 w235 w243 w262]
                tunnel: w220 -> [_ _ _ w261]
                tunnel: [w228 w235 w243 w260] -> w218
                frame " ", Default {
                }
                frame "GPVTG" {
                  (unwired) "$GPVTG,054.7,T,034.4,M,005.5,N,010.2,K*48" ("$GPVTG-message_IN")
                  n163 = call "NMEA_ParseMessage-GPVTG.vi"("$GPVTG-message_IN"=w236) -> ("$GPVTG-message_OUT"=w234:T6)  [unwired: 9 in, 1 out]
                  "$GPVTG-message_OUT" <- w234
                  n164 = Unbundle By Name(w234) -> ("True Course over Ground"=w230:dbl, "Speed over Ground in km/h"=w229:dbl, "Mode"=w233:T7)
                  n165 = Not Equal?(x=w233, y=T7 "N" ("Mode")) -> (x != y?=w231:bool)
                  n166 = case shown="真" w231 {
                    tunnel: w230 -> [_ w237]
                    tunnel: w229 -> [_ w238]
                    frame False {
                    }
                    frame True {
                      "水平运动速度 (km/h)" <- w238
                      "方位角 (deg)" <- w237
                    }
                  }
                }
                frame "GPRMC" {
                  (unwired) "$GPRMC,225446,A,4916.45,N,12311.12,W,000.5,054.7,191194,020.3,E*68" ("$GPRMC-message_IN")
                  n167 = call "NMEA_ParseMessage-GPRMC.vi"("$GPRMC-message_IN"=w244) -> ("$GPRMC-message_OUT"=w242:T5)  [unwired: 9 in, 1 out]
                  "$GPRMC-message_OUT" <- w242
                  n168 = Unbundle By Name(w242) -> ("Validity"=w241:bool, "TimeStamp"=w240:timestamp, "Date Stamp"=w239:timestamp)
                  "定位状态" <- w241
                  n169 = case shown="真" w241 {
                    tunnel: w240 -> [_ w245]
                    tunnel: w239 -> [_ w246]
                    frame False {
                    }
                    frame True {
                      "时间" <- w245
                      "日期" <- w246
                    }
                  }
                }
                frame "GPGGA" {
                  (unwired) "$GPGGA,123519,4807.038,N,01131.000,E,1,08,0.9,545.4,M,46.9,M,,*47" ("data out")
                  n170 = call "NMEA_ParseMessage-GPGGA.vi"("$GPGGA-message_IN"=w265) -> ("$GPGGA-message_OUT"=w252:T2)  [unwired: 9 in, 1 out]
                  "$GPGGA-message_OUT" <- w252
                  n171 = Unbundle By Name(w252) -> ("Horizontal Dilution of Precision"=w253:dbl, "Altitude above Mean-Sea-Level"=w254:dbl, "Latitude-Direction"=w263:T3, "Latitude"=w249:dbl, "Longitude"=w251:dbl, "Longitude-Direction"=w264:T4, "GPS-Quality"=w255:T1)
                  "GPS-Quality" <- w255
                  n172 = global write "NMEA过程全局变量.vi" "GPS$GNGGA-message_OUT"(w252) -> ()
                  n173 = Greater Or Equal?(x=w249, y=1000.0) -> (x >= y?=w247:bool)
                  n174 = Greater Or Equal?(x=w251, y=9000.0) -> (x >= y?=w258:bool)
                  n175 = Equal?(x=w255, y=NMEA_GPS-Quality."GPS fix (SPS)" ("GPS-Quality")) -> (x = y?=w256:bool)
                  n176 = Compound Arithmetic op=AND(w247, w258, w256) -> (w259:bool)
                  n177 = case shown="真" w259 {
                    tunnel: w264 -> [_ w285]
                    tunnel: w249 -> [_ w279]
                    tunnel: w263 -> [_ w278]
                    tunnel: w252 -> [_ w284]
                    tunnel: w262 -> [w266 w283]
                    tunnel: w261 -> [_ w282]
                    tunnel: [w266 w281] -> w260
                    tunnel: w251 -> [_ w280]
                    tunnel: w254 -> [_ w277]
                    tunnel: w253 -> [_ _]
                    frame False {
                    }
                    frame True {
                      n178 = disable-structure shown="禁用" {
                        disable-tunnel: w284 -> [w291 _]
                        disable-tunnel: w283 -> [w290 _]
                        disable-tunnel: w282 -> [w289 _]
                        disable-tunnel: [w287 _] -> w281
                        frame Disabled {
                          n179 = call "NMEA_GPGGA_ToStringArray.vi"("$GPGGA-message_IN"=w291) -> ("$GPGGA-message_OUT"=w288:string[])  [unwired: 9 in, 1 out]
                          n180 = Enqueue Element(queue=w290, element=w288, timeout in ms (-1)=20 ("timeout en ms (-1)"), error in (no error)=w289) -> (queue out=w287:refnum<queue>)  [unwired: 2 out]
                        }
                        frame Enabled {
                        }
                      }
                      n181 = call "NMEA_Coord-ToDecimalDegrees.vi"("Longitude-Direction"=w285, "Latitude-Direction"=w278, "Longitude"=w280, "Latitude"=w279) -> ("Longitude"=w267:dbl, "Latitude"=w268:dbl)  [unwired: 6 in]
                      "经度" <- w267
                      "纬度" <- w268
                      n182 = global read "内部交互全局变量.vi" "其他"() -> (w270:T11)
                      n183 = feedback #1() -> (w273:cluster{"Longitude":dbl, "Latitude":dbl}[])  [unwired: 1 in]
                      n184 = Bundle By Name(cluster=w270, "北斗-GPS.GPS.经度:"=w267, "北斗-GPS.GPS.纬度:"=w268) -> (w269:T11)
                      n185 = Bundle("Longitude"=w267, "Latitude"=w268) -> (w275:cluster{"Longitude":dbl, "Latitude":dbl})  [unwired: 1 in]
                      n186 = Array Subset(array=w273, length=86400 ("长度")) -> (w274:cluster{"Longitude":dbl, "Latitude":dbl}[])  [unwired: 1 in]
                      n187 = Build Array (concatenate)(w275, w273) -> (w276:cluster{"Longitude":dbl, "Latitude":dbl}[])
                      n188 = feedback-in #1(w276) -> ()
                      n189 = global write "内部交互全局变量.vi" "其他"(w269) -> ()
                      n190 = call <vilib>:"Plot XY.vi"("data"=w274, "dimensions (w,h)"=cluster{"width":i16, "height":i16} {"width"=395, "height"=395}) -> ()  [unwired: 13 in, 1 out]
                      "海拔" <- w277
                    }
                  }
                }
              }
            }
            frame -1 {
            }
          }
          n191 = Wait Until Next ms Multiple(millisecond multiple=u32 1 ("n millisecondes")) -> ()  [unwired: 1 out]
        }
        "Raw data GPS" <- w194
      }
      frame True {
      }
    }
    n192 = Wait Until Next ms Multiple(millisecond multiple=u32 1 ("n millisecondes")) -> ()  [unwired: 1 out]
  }
  n193 = while {
    shift-right: [w314] -> _
    shift-left: 0.0 -> [w311]
    shift-right: [w306] -> _
    shift-left: w29 -> [w309]
    shift-right: [w307] -> _
    shift-left: w30 -> [w308]
    stop <- FALSE stop-if-true
    # "Excludes inaccuracy of GPS from processing"
    n194 = local read "经度"() -> (w304:dbl)
    n195 = Wait Until Next ms Multiple(millisecond multiple=u32 1000 ("Refresh period (ms)")) -> ()  [unwired: 1 out]
    n196 = local read "水平运动速度 (km/h)"() -> (w305:dbl)
    n197 = local read "纬度"() -> (w303:dbl)
    n198 = Greater Or Equal?(x=w305, y=0.1) -> (x >= y?=w316:bool)
    n199 = case shown="真" w316 {
      tunnel: w309 -> [_ w327]
      tunnel: w308 -> [_ w325]
      tunnel: w303 -> [_ w324]
      tunnel: w304 -> [_ w326]
      tunnel: w311 -> [w322 _]
      tunnel: [w322 w323] -> w314
      frame False {
      }
      frame True {
        # "Mean radius of the Earth in meters"
        n200 = formula code="lat_new = lat_new*Pi/180;\nlat_old = lat_old*Pi/180;\nlong_new = long_new*Pi/180;\nlong_old = long_old*Pi/180;\nd = asin(sqrt(sin((lat_old-lat_new)/2)**2+cos(lat_new)*cos(lat_old)*sin((long_old-long_new)/2)**2));\nd = 2*d*r/1000;"("Pi"=3.141592653589793, "r"=6372795.0, "long_old"=w327, "long_new"=w326, "lat_old"=w325, "lat_new"=w324) -> ("d"=w323:dbl)
      }
    }
    n201 = case shown="真" "reset odometer" {
      tunnel: w309 -> [w319 _]
      tunnel: w308 -> [w318 _]
      tunnel: w303 -> [_ w320]
      tunnel: w304 -> [_ w321]
      tunnel: [w319 w321] -> w306
      tunnel: [w318 w320] -> w307
      frame False {
      }
      frame True {
      }
    }
    n202 = Multiply(x=1000.0, y=w314) -> (x*y=w302:dbl)
    n203 = Less Or Equal?(x=w302, y=10000.0) -> (x <= y?=w300:bool)
    n204 = Bundle("纬度"=w307, "经度"=w306) -> (→"浮标定位点":cluster{"纬度":dbl, "经度":dbl})  [unwired: 1 in]
    n205 = case shown="真" w300 {
      tunnel: w302 -> [_ w317]
      frame False {
      }
      frame True {
        n206 = global write "NMEA过程全局变量.vi" "GPSOdometer"(w317) -> ()
        "偏移量/米" <- w317
      }
    }
  }
